vi "createEnumArray.vi"(8 "error in (no error)":errorcluster, 10 "enums":string, 11 "Enum in":refnum<class "Enum.lvclass">) -> (0 "error out":errorcluster, 3 "Enum out":refnum<class "Enum.lvclass">)   [LabVIEW 2016, in "Enum.lvclass"]
uses:
  Enum.lvclass
  Enum.lvclass/Enum.ctl
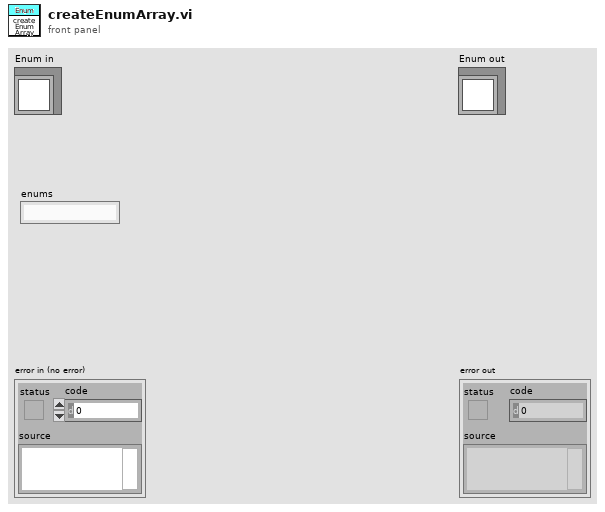
[diagram p1: front panel]
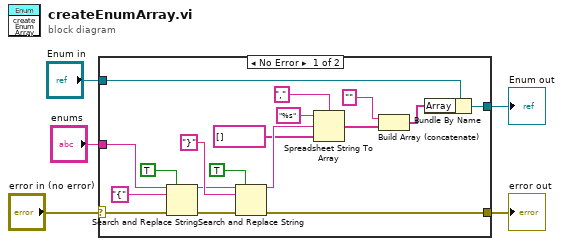
[diagram p0: block diagram]
diagram:
  n1 = case shown="No Error" "error in (no error)" {
    selector: "error in (no error)" -> [w17 w25]
    tunnel: [w11 w25] -> w4
    tunnel: [w9 w24] -> w2
    tunnel: "Enum in" -> [w10 w24]
    tunnel: "enums" -> [w23 _]
    frame No Error {
      n2 = Search and Replace String(replace all?=TRUE ("replace all? (F)"), input string=w23, search string="{", error in=w17) -> (result string=w18:string, error out=w16:errorcluster)  [unwired: 4 in, 2 out]
      n3 = Search and Replace String(replace all?=TRUE ("replace all? (F)"), input string=w18, search string="}", error in=w16) -> (result string=w14:string, error out=w11:errorcluster)  [unwired: 4 in, 2 out]
      n4 = Spreadsheet String To Array(delimiter (Tab)=",", format string="%s", spreadsheet string=w14, array type (2D Dbl)=string[] []) -> (array=w7:string[])
      n5 = Build Array (concatenate)("" ("format string"), w7) -> (w8:string[])
      n6 = Bundle By Name(cluster=w10, "Array"=w8) -> (w9:refnum<class "Enum.lvclass">)
    }
    frame Error {
    }
  }
  "error out" <- w4
  "Enum out" <- w2
